vi "fill.vi"(8 "error in (no error)":errorcluster, 10 "value":u8, 11 "Image in":T1) -> (0 "error out":errorcluster, 3 "Image out":T1)   [LabVIEW 2022 SP3, in "Vision.lvlib"]
uses:
  Vision.lvlib
  <vilib>/vision/Image Controls.llb/IMAQ Image.ctl
  bin/Vision.dll
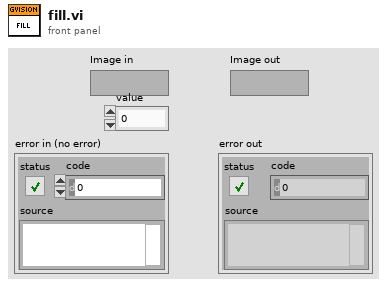
[diagram p1: front panel]
types:
  T1 = typedef "IMAQ Image.ctl" = refnum<image>
  T2 = enum32{"Map Pixel Pointer", "Unmap Pixel Pointer", "Get Pixels Infos"}
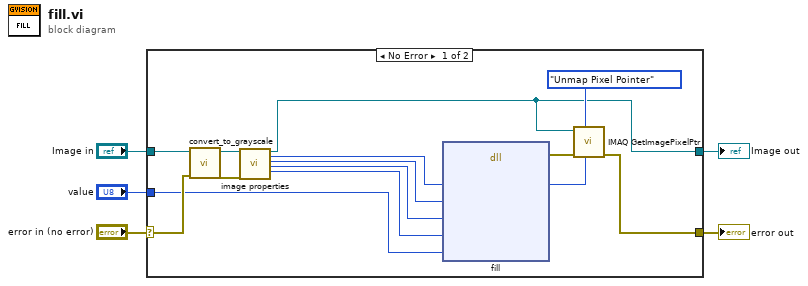
[diagram p0: block diagram]
diagram:
  n1 = case shown="No Error" "error in (no error)" {
    selector: "error in (no error)" -> [w16 w21]
    tunnel: "Image in" -> [w17 w20]
    tunnel: [w6 w21] -> w3
    tunnel: [w7 w20] -> w2
    tunnel: "value" -> [w9 _]
    frame No Error {
      n2 = call "convert_to_grayscale.vi"("error in (no error)"=w16, "Image in"=w17) -> ("error out"=w14:errorcluster, "Image out"=w15:T1)  [unwired: 8 in]
      n3 = call "image properties.vi"("Image in"=w15, "error in (no error)"=w14) -> ("Image out"=w7:T1, "Pixel Pointer out"=w13:u64, "Line Width"=w12:i32, "X Resolution"=w11:i32, "Y Resolution"=w10:i32)  [unwired: 11 in, 2 out]
      n4 = dll-call lib="C:/Users/Caleb/Desktop/nebraska-silicon-lab/pixel-gantry-control/Gantry/Shared Components/External/bin/Vision.dll" fn="fill"("src_imgPtr"=w13, "src_imgLineWidth"=w12, "src_imgWidth"=w11, "src_imgHeight"=w10, "value"=w9) -> (error out=w19:errorcluster, "src_imgPtr"=w8:u64)  [unwired: 8 in, 1 out]
      n5 = call "IMAQ GetImagePixelPtr"("Pixel Pointer in"=w8, "Function"=T2."Unmap Pixel Pointer", "error in (no error)"=w19, "Image"=w7) -> ("error out"=w6:errorcluster)  [unwired: 2 in, 5 out]
    }
    frame Error {
    }
  }
  "Image out" <- w2
  "error out" <- w3
